vi "QSM - Add State(s).vi"   [LabVIEW 2014]
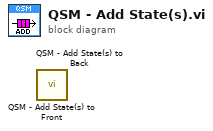
[diagram p0: block diagram]
diagram:
  n1 = call "QSM - Add State(s) to Front.vi"() -> ()  [unwired: 11 in, 1 out]
  n2 = call "QSM - Add State(s) to Back.vi"() -> ()  [unwired: 11 in, 1 out]
